vi "IMAQ-MWT HT TEST (HOST).vi"() -> ()   [LabVIEW 2015]
uses:
  <vilib>/Analysis/baseanly.llb/Mean (DBL).vi
  <vilib>/FPGAPlugInAG/PCIe-1473R-LX110/niLvFpga_Open_PCIe-1473R-LX110.vi
  <vilib>/rvi/interface/common/dynamic/niFpgaDynamicAddResources.vi
  <vilib>/rvi/interface/common/niFpgaWaitOnOcc.vi
  <vilib>/Utility/error.llb/Error Cluster From Error Code.vi
  <vilib>/rvi/errors/niLvFpgaAdjustHostInterfaceError.vi
  <vilib>/FPGAPlugInAG/Dynamic/niLvFpga_Close_Dynamic.vi
  <vilib>/rvi/interface/nirviOpenFPGA/nirviOpenFPGA.xnode
  FPGA Bitfiles/IMAQ-MWT HT TEST (FPGA) (with Angle Sorting).lvbitx
  <vilib>/rvi/interface/nirviMethod/nirviMethod.xnode
  <vilib>/rvi/interface/nirviReadWriteControl/nirviReadWriteControl.xnode
  <vilib>/rvi/interface/nirviCloseFPGA/nirviCloseFPGA.xnode
  NiFpgaLv.dll
  <vilib>/rvi/interface/Simulation/niFpgaSimulationCallBeginRW.vi
  <vilib>/rvi/errors/niLvFpgaMergeErrorWithErrorCode.vi
  <vilib>/FPGAPlugInAG/Dynamic/niLvFpga_ReadFifo_Dynamic.vi
  <vilib>/Analysis/NI_AALBase.lvlib
  <vilib>/FPGAPlugInAG/Dynamic/niLvFpga_WriteFifo_Dynamic.vi
  <vilib>/FPGAPlugInAG/Dynamic/niLvFpga_ConfigureFifo_Dynamic.vi
  <vilib>/FPGAPlugInAG/Dynamic/niLvFpga_StartFifo_Dynamic.vi
panel:
  out "Angle 2":fxp<+/-,16,3> format="%.14g"
  out "Angle 1":fxp<+/-,16,3> format="%.14g"
  out "Mean Angle":fxp<+/-,32,16> format="%.21g"
  out "Valleys":u64[](graph)
  out "Peaks":u64[](graph)
  out "Angle":dbl[](graph)
  in  "Frame # Processing":i32=40
  out "Frame #":i32
  in  "Loop Interval":u32=1000
  in  "Stop Button":bool
  out "N Points":u16
  out "V2 (ID)":i32
  out "V1 (ID)":i32
  out "SPLINE":cluster{u16[], u16[]}[](graph)
  out "Contour":cluster{u16[], u16[]}(graph)
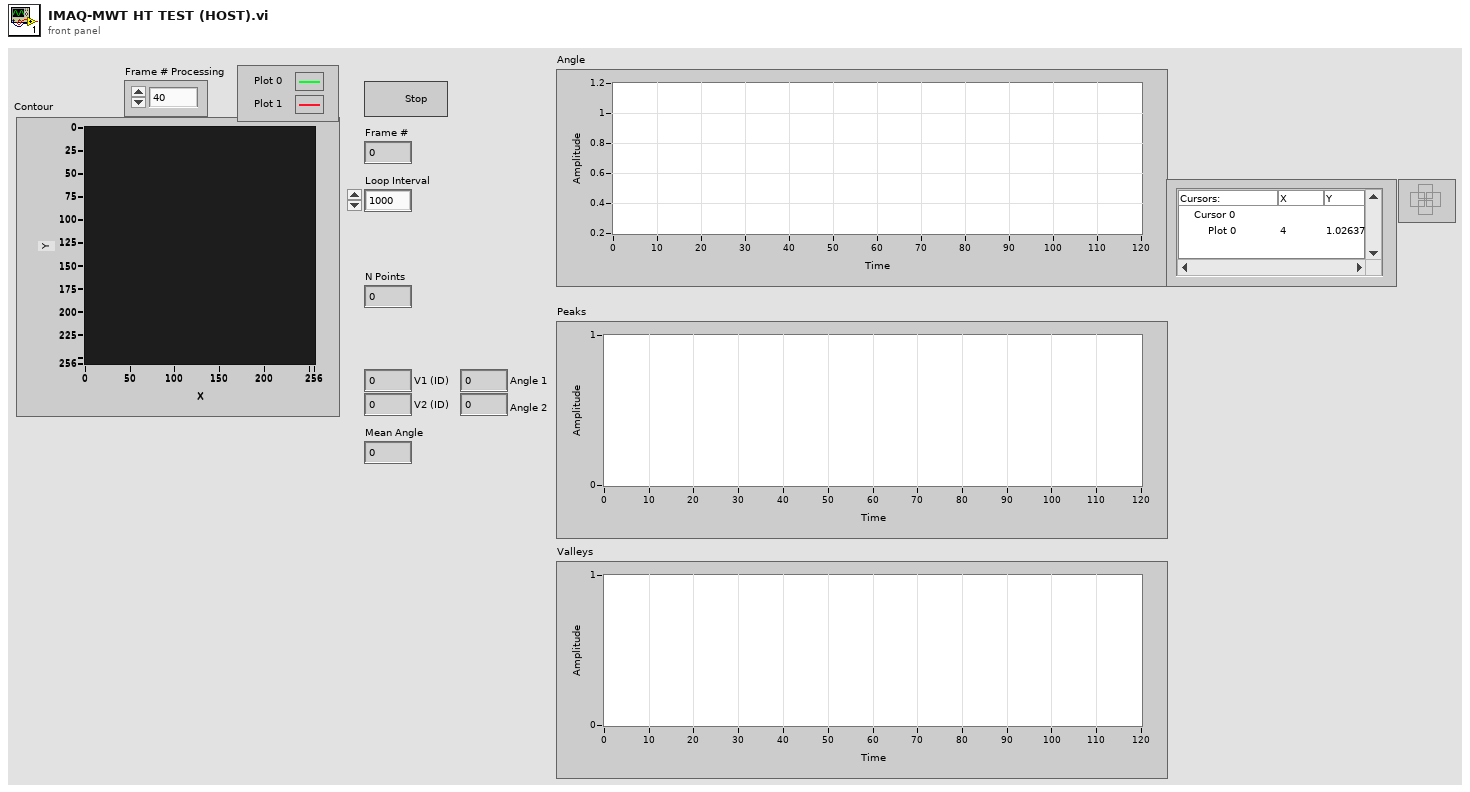
[diagram p1: front panel]
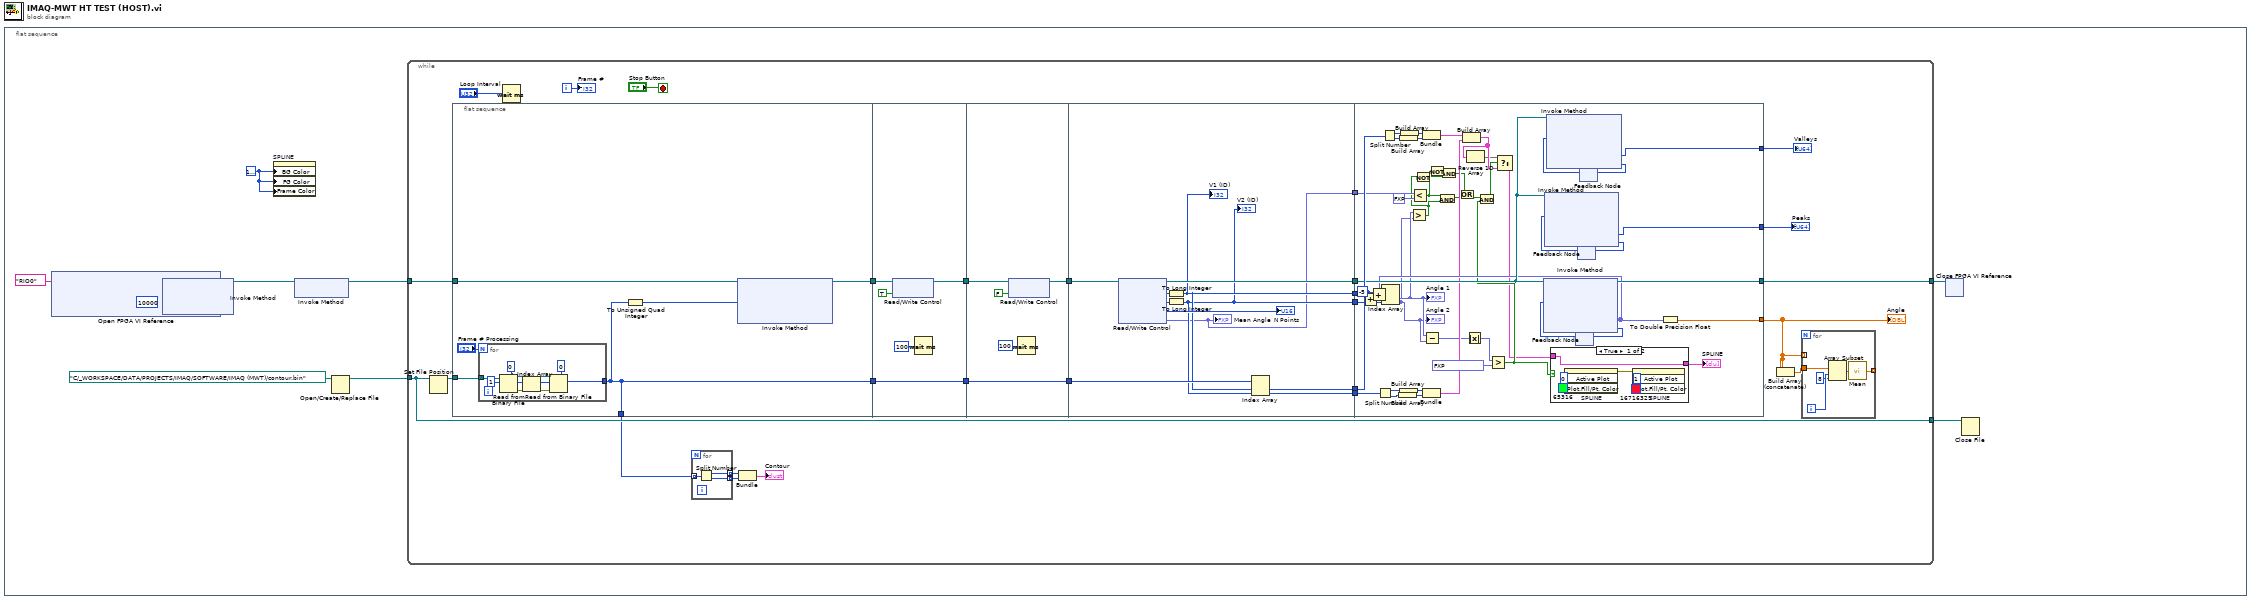
[diagram p0: block diagram]
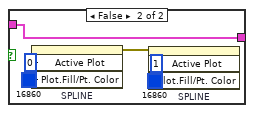
[diagram p2: hidden frame]
diagram:
  n1 = flat-sequence {
    frame #0 {
      w5 = u32 16777216 ("Plot Area:Colors:BG Color")
      n2 = xnode "Open FPGA VI Reference"("resource name"=tag "RIO0") -> ("FPGA VI Reference Out"=w4:refnum<k20>)  [unwired: 1 in, 1 out]
      n3 = xnode "Invoke Method"("FPGA VI Reference In"=w4, "Requested Depth"=u32 10000) -> ("FPGA VI Reference Out"=w2:refnum<k20>)  [unwired: 1 in, 2 out]
      n4 = property on="SPLINE" class="XYGraph (strict)"("BG Color"=w5, "FG Color"=w5, "Frame Color"=w5) -> ()  [unwired: 2 in, 2 out]
      n5 = xnode "Invoke Method"("FPGA VI Reference In"=w2) -> ("FPGA VI Reference Out"=w1:refnum<k20>)  [unwired: 1 in, 1 out]
      n6 = Open/Create/Replace File(file path (use dialog)=path "C:/_WORKSPACE/DATA/PROJECTS/IMAQ/SOFTWARE/IMAQ (MWT)/contour.bin") -> (refnum out=w8:refnum<file>)  [unwired: 5 in, 2 out]
      n7 = while {
        tunnel: w1 -> [w37]
        tunnel: [w33] -> w9
        tunnel: w8 -> [w31]
        tunnel: [w31] -> w7
        i -> [w24]
        stop <- "Stop Button" stop-if-true
        n8 = Set File Position(refnum=w31) -> (refnum out=w18:refnum<file>)  [unwired: 3 in, 1 out]
        n9 = flat-sequence {
          tunnel: w37 -> [w51]
          tunnel: [w50] -> w36
          tunnel: w18 -> [w49]
          tunnel: [w47] -> w26
          tunnel: [w47] -> w21
          tunnel: w36 -> [w65]
          tunnel: [w63] -> w35
          tunnel: [w61] -> w22
          tunnel: w21 -> [w61]
          tunnel: w35 -> [w70]
          tunnel: [w69] -> w34
          tunnel: [w66] -> w23
          tunnel: w22 -> [w66]
          tunnel: w34 -> [w81]
          tunnel: [w80] -> w25
          tunnel: w23 -> [w78]
          tunnel: [w75] -> w20
          tunnel: [w74] -> w19
          tunnel: [w73] -> w13
          tunnel: [w72] -> w12
          tunnel: [w71] -> w11
          tunnel: [w128] -> w33
          tunnel: w25 -> [w119]
          tunnel: w20 -> [w130]
          tunnel: w19 -> [w129]
          tunnel: [w118] -> w14
          tunnel: [w123] -> w17
          tunnel: [w122] -> w16
          tunnel: w13 -> [w116]
          tunnel: w12 -> [w115]
          tunnel: w11 -> [w92]
          frame #0 {
            n10 = for {
              N: "Frame # Processing" -> [_]
              tunnel: w49 -> [w60]
              tunnel: [w52] -> w47
              n11 = Read from Binary File(5:0 ("count (1)"), 10:1 ("count (1)"), 11:w60) -> (0:w58:errorcluster, 2:w55:i32[], 3:w57:refnum<file>)  [unwired: 3 in, 1 out]
              n12 = Index Array(array=w55) -> (element=w54:i32)  [unwired: 1 in]
              n13 = Read from Binary File(5:u32 0 ("count (1)"), 8:w58, 10:w54, 11:w57) -> (2:w52:u32[])  [unwired: 2 in, 3 out]
            }
            n14 = To Unsigned Quad Integer(1:w47) -> (0:w46:u64[])
            n15 = xnode "Invoke Method"("FPGA VI Reference In"=w51, "Data"=w46) -> ("FPGA VI Reference Out"=w50:refnum<k20>)  [unwired: 2 in, 2 out]
          }
          frame #1 {
            n16 = xnode "Read/Write Control"("FPGA VI Reference In"=w65, "Scan End?"=TRUE) -> ("FPGA VI Reference Out"=w63:refnum<k20>)  [unwired: 1 in, 1 out]
            n17 = Wait (ms)(milliseconds to wait=u32 100) -> ()  [unwired: 1 out]
          }
          frame #2 {
            n18 = xnode "Read/Write Control"("FPGA VI Reference In"=w70, "Scan End?"=FALSE) -> ("FPGA VI Reference Out"=w69:refnum<k20>)  [unwired: 1 in, 1 out]
            n19 = Wait (ms)(milliseconds to wait=u32 100) -> ()  [unwired: 1 out]
          }
          frame #3 {
            n20 = xnode "Read/Write Control"("FPGA VI Reference In"=w81) -> ("FPGA VI Reference Out"=w80:refnum<k20>, "V1 (ID)"=w77:u16, "V2 (ID)"=w76:u16, "N Points"=→"N Points":u16, "Mean Angle"=w71:fxp<+/-,32,16>)  [unwired: 1 in, 1 out]
            "Mean Angle" <- w71
            n21 = To Long Integer(number=w77) -> (32bit integer=w73:i32)
            "V1 (ID)" <- w73
            n22 = To Long Integer(number=w76) -> (32bit integer=w72:i32)
            "V2 (ID)" <- w72
            n23 = Index Array(array=w78, index #1=w73, index #2=w72) -> (element #1=w75:u32, element #2=w74:u32)
          }
          frame #4 {
            w99 = -5 ("x")
            n24 = Add(x=w99, y=w115) -> (x+y=w100:i32)
            n25 = Add(x=w99, y=w116) -> (x+y=w101:i32)
            n26 = Split Number(x=w129) -> (hi(x)=w111:u16, lo(x)=w112:u16)
            n27 = Split Number(x=w130) -> (hi(x)=w114:u16, lo(x)=w113:u16)
            n28 = Build Array(w112) -> (w105:u16[])
            n29 = Build Array(w113) -> (w107:u16[])
            n30 = Build Array(w111) -> (w106:u16[])
            n31 = Build Array(w114) -> (w108:u16[])
            n32 = Less?(x=w92, y=fxp<+/-,32,16> 1.0) -> (x < y?=w91:bool)
            n33 = Bundle(w108, w107) -> (w109:cluster{u16[], u16[]})  [unwired: 1 in]
            n34 = Bundle(w106, w105) -> (w110:cluster{u16[], u16[]})  [unwired: 1 in]
            n35 = Not(x=w91) -> (.not. x?=w90:bool)
            n36 = Build Array(w109, w110) -> (w85:cluster{u16[], u16[]}[])
            n37 = Reverse 1D Array(array=w85) -> (reversed array=w84:cluster{u16[], u16[]}[])
            n38 = feedback #1() -> (w126:u32)  [unwired: 1 in]
            n39 = xnode "Invoke Method"("FPGA VI Reference In"=w119, "Number of Elements"=w126) -> ("FPGA VI Reference Out"=w128:refnum<k20>, "Data"=w117:fxp<+/-,16,3>[], "Elements Remaining"=w127:u32)  [unwired: 2 in, 1 out]
            n40 = Index Array(array=w117, index #1=w101, index #2=w100) -> (element #1=w98:fxp<+/-,16,3>, element #2=w97:fxp<+/-,16,3>)
            "Angle 1" <- w98
            "Angle 2" <- w97
            n41 = Greater?(x=w98, y=w97) -> (0:w88:bool)
            n42 = Not(x=w88) -> (.not. x?=w89:bool)
            n43 = Subtract(x=w98, y=w97) -> (x-y=w104:fxp<+/-,17,4>)
            n44 = And(x=w91, y=w88) -> (x .and. y?=w94:bool)
            n45 = And(x=w90, y=w89) -> (x .and. y?=w87:bool)
            n46 = Or(x=w87, y=w94) -> (x .or. y?=w93:bool)
            n47 = Absolute Value(x=w104) -> (abs(x)=w103:fxp<+,16,3>)
            n48 = Greater?(x=w103, y=fxp<+,16,3> 0.050048828125) -> (0:w95:bool)
            n49 = And(x=w93, y=w95) -> (x .and. y?=w86:bool)
            n50 = Select(t=w84, s=w86, f=w85) -> (s? t:f=w83:cluster{u16[], u16[]}[])
            n51 = case shown="True" w95 {
              tunnel: w83 -> [w131 w138]
              tunnel: [w131 w138] -> w82
              frame True {
                n52 = property on="SPLINE" class="XYGraph (strict)"("Active Plot"=u32 0, "Plot.Fill/Pt. Color"=u32 65316) -> (error out=w132:errorcluster)  [unwired: 2 in, 1 out]
                n53 = property on="SPLINE" class="XYGraph (strict)"(error in=w132, "Active Plot"=u32 1, "Plot.Fill/Pt. Color"=u32 16716329) -> ()  [unwired: 1 in, 2 out]
              }
              frame False {
                n54 = property on="SPLINE" class="XYGraph (strict)"("Active Plot"=u32 0, "Plot.Fill/Pt. Color"=u32 16860) -> (error out=w139:errorcluster)  [unwired: 2 in, 1 out]
                n55 = property on="SPLINE" class="XYGraph (strict)"(error in=w139, "Active Plot"=u32 1, "Plot.Fill/Pt. Color"=u32 16860) -> ()  [unwired: 1 in, 2 out]
              }
            }
            "SPLINE" <- w82
            n56 = feedback-in #1(w127) -> ()
            n57 = feedback #2() -> (w125:u32)  [unwired: 1 in]
            n58 = xnode "Invoke Method"("FPGA VI Reference In"=w119, "Number of Elements"=w125) -> ("Data"=w123:u64[], "Elements Remaining"=w124:u32)  [unwired: 2 in, 2 out]
            n59 = feedback-in #2(w124) -> ()
            n60 = feedback #3() -> (w120:u32)  [unwired: 1 in]
            n61 = xnode "Invoke Method"("FPGA VI Reference In"=w119, "Number of Elements"=w120) -> ("Data"=w122:u64[], "Elements Remaining"=w121:u32)  [unwired: 2 in, 2 out]
            n62 = feedback-in #3(w121) -> ()
            n63 = To Double Precision Float(number=w117) -> (double precision float=w118:dbl[])
          }
        }
        n64 = Wait (ms)(milliseconds to wait="Loop Interval") -> ()  [unwired: 1 out]
        n65 = for {
          tunnel: w26 -> [w45] mode=indexing
          tunnel: [w44] -> w28 mode=indexing
          tunnel: [w43] -> w29 mode=indexing
          n66 = Split Number(x=w45) -> (hi(x)=w44:u16, lo(x)=w43:u16)
        }
        n67 = Bundle(w28, w29) -> (→"Contour":cluster{u16[], u16[]})  [unwired: 1 in]
        n68 = Build Array (concatenate)(w14, w14) -> (w15:dbl[])
        n69 = for {
          tunnel: w14 -> [_] mode=indexing
          tunnel: w15 -> [w42]
          tunnel: [w38] -> _ mode=indexing
          i -> [w41]
          n70 = Array Subset(array=w42, index=w41, length=8) -> (w39:dbl[])
          n71 = call-poly <vilib>:"Mean.vi"("X"=w39) -> ("mean"=w38:dbl)  [unwired: 1 out]
        }
        "Frame #" <- w24
        "Angle" <- w14
        "Peaks" <- w17
        "Valleys" <- w16
      }
      n72 = xnode "Close FPGA VI Reference"("FPGA VI Reference In"=w9) -> ()  [unwired: 1 in, 1 out]
      n73 = Close File(refnum=w7) -> ()  [unwired: 1 in, 2 out]
    }
  }
